vi "expand string for MUX80 config.vi"(7 "RegEx":string, 8 "Input Config Str":string, 9 "Default Config Str":string, 11 "NumChannels":i32) -> (0 "Good Initial Arr":bool, 2 "Output Config Arr":string[](array[string]))   [LabVIEW 2020]
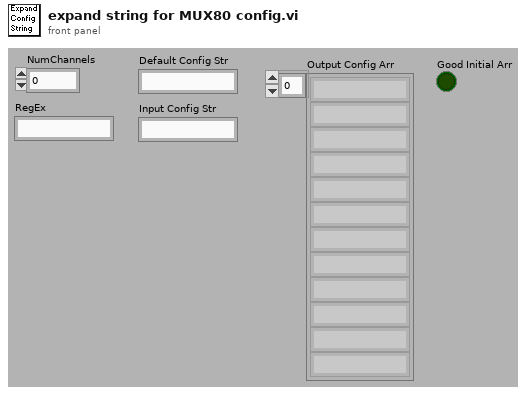
[diagram p1: front panel]
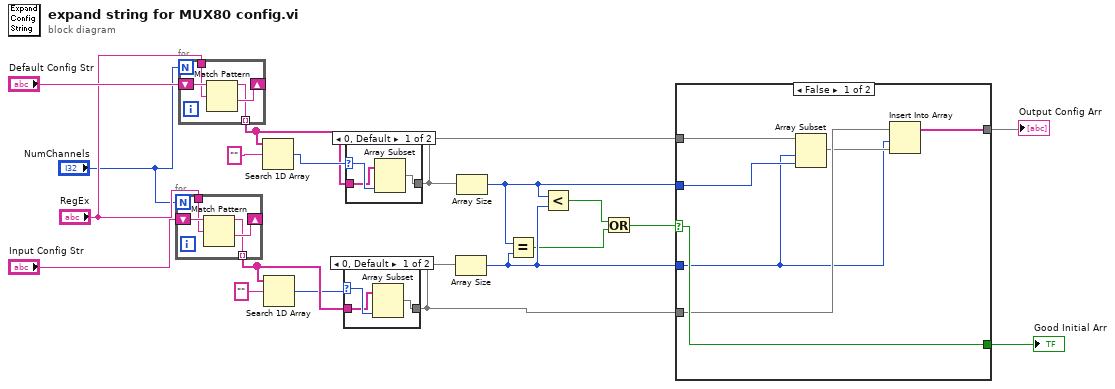
[diagram p0: block diagram]
diagram:
  n1 = for {
    N: "NumChannels" -> [_]
    shift-right: [w21] -> _
    shift-left: "Input Config Str" -> [w23]
    tunnel: "RegEx" -> [w22]
    tunnel: [w20] -> w2 mode=indexing
    n2 = Match Pattern(string=w23, regular expression=w22) -> (before substring=w20:string, after substring=w21:string)  [unwired: 1 in, 2 out]
  }
  n3 = for {
    N: "NumChannels" -> [_]
    shift-right: [w25] -> _
    shift-left: "Default Config Str" -> [w27]
    tunnel: "RegEx" -> [w26]
    tunnel: [w24] -> w5 mode=indexing
    n4 = Match Pattern(string=w27, regular expression=w26) -> (before substring=w24:string, after substring=w25:string)  [unwired: 1 in, 2 out]
  }
  n5 = Search 1D Array(1D array=w5, element="") -> (index of element=w6:i32)  [unwired: 1 in]
  n6 = Search 1D Array(1D array=w2, element="") -> (index of element=w1:i32)  [unwired: 1 in]
  n7 = case shown="0, Default" w1 {
    selector: w1 -> [w30 _]
    tunnel: w2 -> [w29 w31]
    tunnel: [w28 w31] -> w3
    frame 0, Default {
      n8 = Array Subset(array=w29, length=w30) -> (w28:string[])  [unwired: 1 in]
    }
    frame -1 {
    }
  }
  n9 = case shown="0, Default" w6 {
    selector: w6 -> [w34 _]
    tunnel: w5 -> [w33 w35]
    tunnel: [w32 w35] -> w4
    frame 0, Default {
      n10 = Array Subset(array=w33, length=w34) -> (w32:string[])  [unwired: 1 in]
    }
    frame -1 {
    }
  }
  n11 = Array Size(array=w3) -> (size(s)=w18:i32)
  n12 = Array Size(array=w4) -> (size(s)=w14:i32)
  n13 = Equal?(x=w14, y=w18) -> (x = y?=w16:bool)
  n14 = Less?(x=w14, y=w18) -> (x < y?=w17:bool)
  n15 = Or(x=w17, y=w16) -> (x .or. y?=w15:bool)
  n16 = case shown="False" w15 {
    selector: w15 -> [w42 w44]
    tunnel: [w42 w44] -> w19
    tunnel: w4 -> [w41 _]
    tunnel: w3 -> [w40 w43]
    tunnel: w18 -> [w36 _]
    tunnel: w14 -> [w37 _]
    tunnel: [w38 w43] -> w13
    frame False {
      n17 = Array Subset(array=w41, index=w36, length=w37) -> (w39:string[])
      n18 = Insert Into Array(array=w40, index=w36, new element=w39) -> (w38:string[])
    }
    frame True {
    }
  }
  "Good Initial Arr" <- w19
  "Output Config Arr" <- w13
